vi "StopHarvest.vi"(8 "Error in":errorcluster, 11 "Controller in":refnum<class "Controller.lvclass">) -> (0 "Error out":errorcluster, 3 "Controller out":refnum<class "Controller.lvclass">, 10 "StopHarvest":cluster{"Stop":bool})   [LabVIEW 2021, in "Controller.lvlib" / "Controller.lvclass"]
uses:
  Controller.lvclass
  Controller.lvclass/Controller.ctl
  <vilib>/ActorFramework/Message Enqueuer/Message Enqueuer.lvclass/Message Enqueuer.ctl
  UserInterface/UserInterface Messages/Log Data Msg/Log Data Msg.lvclass/Log Data Msg.ctl
  <vilib>/ActorFramework/Message Enqueuer/Enqueue.vi
  PLCHandler/PLCHandler Messages/Sleep Msg/Sleep Msg.lvclass
  C:/Program Files/National Instruments/LabVIEW 2021/vi.lib/ActorFramework/Message/Message.lvclass
  UserInterface/UserInterface Messages/Log Data Msg/Log Data Msg.lvclass
  <vilib>/ActorFramework/Message Priority Queue/Priority Enqueue.vi
  <vilib>/ActorFramework/Message Enqueuer/Message Enqueuer.lvclass
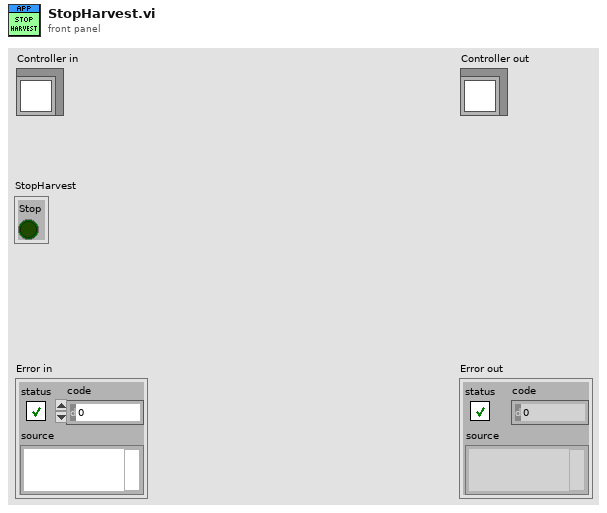
[diagram p1: front panel]
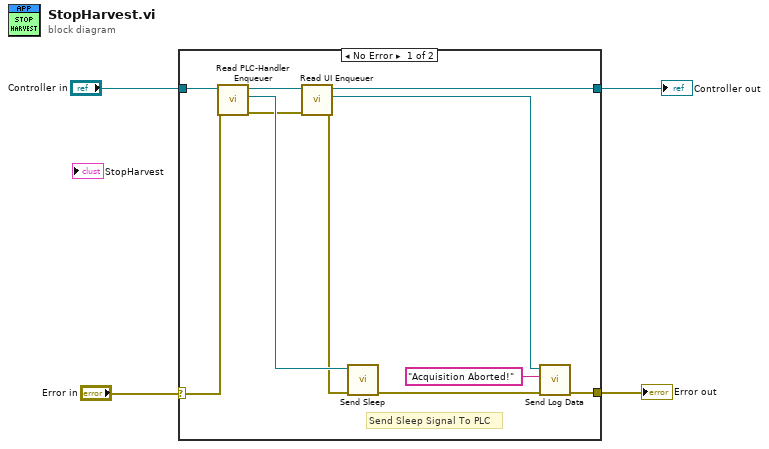
[diagram p0: block diagram]
diagram:
  n1 = case shown="No Error" "Error in" {
    selector: "Error in" -> [w14 w16]
    tunnel: "Controller in" -> [w15 w17]
    tunnel: [w11 w17] -> w2
    tunnel: [w8 w16] -> w1
    frame No Error {
      # "Send Sleep Signal To PLC"
      n2 = call "Read PLC-Handler Enqueuer.vi"("error in (no error)"=w14, "Controller in"=w15) -> ("error out"=w7:errorcluster, "Actor Framework:Message Enqueuer"=w13:refnum<class "Message Enqueuer.lvclass">, "Controller out"=w12:refnum<class "Controller.lvclass">)  [unwired: 7 in]
      n3 = call "Read UI Enqueuer.vi"("error in (no error)"=w7, "Controller in"=w12) -> ("error out"=w6:errorcluster, "Actor Framework:Message Enqueuer"=w10:refnum<class "Message Enqueuer.lvclass">, "Controller out"=w11:refnum<class "Controller.lvclass">)  [unwired: 7 in]
      n4 = call "Send Sleep.vi"("error in (no error)"=w6, "Message Enqueuer"=w13) -> ("error out"=w9:errorcluster)  [unwired: 8 in, 1 out]
      n5 = call "Send Log Data.vi"("error in (no error)"=w9, "Message"="Acquisition Aborted!", "Message Enqueuer"=w10) -> ("error out"=w8:errorcluster)  [unwired: 7 in, 1 out]
    }
    frame Error {
    }
  }
  "Error out" <- w1
  "Controller out" <- w2
